vi "main.vi"() -> ()   [LabVIEW 2013]
uses:
  <vilib>/userdefined/High Color/IMAQdx.ctl
  <vilib>/Analysis/baseanly.llb/Mean (DBL).vi
  <vilib>/DAQmx/read.llb/DAQmx Read (Analog 1D Wfm NChan NSamp).vi
  <vilib>/measure/mascope.llb/Amplitude and Levels 1 chan.vi
  <vilib>/measure/mamon.llb/Trigger Detection for 1 Channel.vi
  <vilib>/Waveform/WDTOps.llb/WDT Append Waveforms DBL.vi
  <vilib>/DAQmx/miscellaneous.llb/DAQmx Fill In Error Info.vi
  <vilib>/measure/NI_MAPro.lvlib
  <vilib>/Analysis/NI_AALBase.lvlib
  <vilib>/vision/driver/NI_Vision_Acquisition_Software.lvlib
panel:
  in  "탭 컨트롤":T1(tab)
  out "웨이브폼 차트 2":dbl(graph)
  in  "reset":bool
  out "right":dbl(slide) scale=0.0..0.5
  out "left":dbl(slide)
  out "rear":dbl(slide) scale=0.0..0.5
  out "front":dbl(slide)
  out "trigger":bool
  in  "Force cal val":bool
  out "Triggered Force graph":waveform(dbl)(graph)={"t0"=timestamp(0 s since 1904-01-01), "dt"=0.00062, "Y"=array[3100 elements]}
  out "bonding force":dbl=1.1386680148675508 caption="Bonding force (kg)" format="%.3f"
  out "Bondtime":dbl=0.5053000000000001 caption="Bonding time" format="%.3f"
  out "vacum":dbl=1.2177873383633695 format="%#_3f"
  out "Heater temp":dbl=nan format="%0.2f"
  out "2":dbl(slide)
  out "슬라이드":dbl(slide)
  out "슬라이드 2":dbl(slide) scale=0.0..1.0
  out "슬라이드 3":dbl(slide) scale=0.0..1.0
  out "XY 그래프":cluster{dbl[], dbl[]}(graph)
  out "vaccum 차트 3":waveform(dbl)(graph)={"t0"=timestamp(3477442777.176875 s since 1904-01-01), "dt"=0.01, "Y"=[0.9261417940939543, 0.9261417940939543, 0.9261417940939543, 0.9261417940939543, 0.9261417940939543, 0.9261417940939543, 0.9261417940939543, 0.9261417940939543, 0.9261417940939543, 0.9261417940939543], "attributes"=variant("NI_ChannelName"=variant(string "전압"), "NI_UnitDescription"=variant(string "Volts"))}
  out "Force raw chart":waveform(dbl)[](graph)=[{"t0"=timestamp(3477442777.13187 s since 1904-01-01), "dt"=0.00062, "Y"=[-1.6112136636470233e-05, -8.569886798010926e-06, -1.9875060209823524e-07, 2.38297423695265e-06, -2.5658168581669667e-06, -1.772821098699811e-06, -4.127955201515539e-06, 6.359857628775875e-07, 4.928880013384412e-07, -3.030881455329775e-06, -1.6476111269731543e-06, -3.5257574105908386e-06, 3.9272455815972755e-06, 4.1657435117466915e-06, 1.9357923056845556e-06, -8.873963893666015e-06, -7.478785108954976e-06, 2.961286460921625e-07, 1.4110617831093333e-07, -1.8980310390713461e-06, 1.6734457588159683e-06, -1.091306434532689e-05, -1.0513727362142483e-06, -6.190924313818898e-06, -1.2540761368932031e-05, -2.1656959207560037e-05, -7.4907097304474685e-06, -3.2872630354662113e-06, -7.950263527933837e-08, -5.964355867846931e-06, -2.4107952296524134e-06, -3.7881010918357573e-06, 2.609546568115507e-06, 1.715182700246618e-06, -5.290612250873919e-06, -6.512889823589868e-06, -3.120361442334684e-07, 5.578846081749961e-06, 7.045614998740958e-06, -1.4627773018794912e-06, -7.937882831116044e-06, -2.595628704294203e-06, 1.2799261966089874e-06, 3.3190306855961753e-07, -3.4363220332503078e-06, -9.953137975658443e-06, 2.3591245238553327e-06, -1.0871470597100204e-06, 8.685197127258367e-07, -7.478785108954976e-06, -8.659321257106097e-06, -4.879210834785539e-06, -3.710590473067321e-06, -4.771888670569855e-06, -1.2516912366543758e-05, -5.576804340679935e-06, -6.274396873296863e-06, -8.546139112344271e-07, 2.2696881098723825e-06, -3.585380986597095e-06, -7.890184386099151e-06, 4.034519211733817e-07, 2.055040781583931e-06, 3.3071514956147953e-06, -2.7625750097582926e-06, -6.900440625190667e-06, 4.2909549706155075e-06, 9.830102788370948e-06, 3.032879356729265e-06, 4.088231671969834e-06, -9.488079817087242e-06, -5.111742111559042e-06, 2.567809552028929e-06, -4.688415860253707e-06, -1.833603522524735e-05, -9.50012139076079e-07, 3.3250388142463035e-06, -2.6135158111173114e-06, -6.769269618278701e-06, -2.0929577385222132e-05, -7.305878065355784e-06, -1.8562943957647073e-06, -3.090505090348801e-06, -3.5257574105908386e-06, -4.932871908254762e-06, -1.033522309183479e-07, -4.169691655199052e-06, 1.94771715199473e-06, -5.254838228130094e-06, -5.147516144541169e-06, 1.2978134427175586e-06, 9.126526251121246e-06, 1.5422725370008507e-06, -4.688415860253707e-06, -2.005353820147982e-06, 4.4518875659287035e-07, 1.7688444872052448e-06, -1.1229213806461855e-06, -6.51885214588969e-06, -1.4490413466475015e-05], "attributes"=variant("NI_ChannelName"=variant(string "변형률_0"), "NI_UnitDescription"=variant(string "Strain"))}, {"t0"=timestamp(3477442777.13187 s since 1904-01-01), "dt"=0.00062, "Y"=[-1.5926450874775857e-06, 1.7934307923881257e-06, -2.236473822173629e-06, -4.09045749208906e-06, -3.881810155491518e-06, 1.7218937409129746e-06, 3.9872386740088464e-06, 1.7192680555871353e-07, 2.2286147427125606e-06, -1.3005373326004466e-06, 3.456670124526979e-06, 8.523920832607e-06, 5.322604705970085e-06, 3.104945216654824e-06, 2.639953345335169e-06, 6.449322569493326e-06, 1.898110120282012e-07, -2.9306233811443237e-07, -7.929552945691535e-06, 2.53892933758521e-05, 6.6698972632327115e-06, 5.113953528386892e-06, 2.425341858268832e-06, -5.911320745626876e-07, -2.8385721664852527e-06, 1.0303694376600552e-06, -3.2286931975534613e-07, -4.793896442446842e-06, -2.7789585013682837e-06, -2.254357941858881e-06, 4.482039064584e-06, 3.188405341896096e-06, 2.890333530003795e-06, 1.5370897386411374e-06, 1.3224787249476363e-06, 5.0603003825103886e-06, 4.470116157849115e-06, 2.0378491288205883e-06, 3.087060905915481e-06, 4.237619533343155e-06, 6.22874797305966e-06, 2.4551490037417866e-06, 8.455656909807571e-07, -1.976799849226179e-07, -2.862417630541878e-06, 5.030493081733363e-06, 2.8068734545164028e-06, -7.640124402846258e-07, -2.105323591603382e-06, 2.3750223240719277e-07, 6.884510572159387e-06, -7.878580032793122e-07, -5.163499562134611e-06, -6.391533772034915e-06, -2.6835766223972933e-06, 4.684728522578421e-06, 2.885317683250044e-08, -1.2826531787987904e-06, -2.8206880676963555e-06, 3.7726266086577194e-06, 6.7414350226397595e-06, 3.3195569954219583e-06, 2.017338166964026e-07, 2.7114905281608864e-06, 3.40301715648635e-06, 9.60891530636603e-06, -7.029395011258529e-06, 2.153804825353152e-05, 1.1194680695472973e-05, -9.786224662971449e-07, 8.702765913475292e-06, -2.558387878634849e-06, -5.911320745626876e-07, -2.4272377325028147e-06, 2.8307191889483254e-06, 5.656446771208991e-06, 1.9901577367198323e-06, -2.2960875519699664e-06, -4.656785538247539e-06, -2.898185824494624e-06, 7.501831387741804e-07, -3.983153158427838e-06, -1.610529230191517e-06, -2.8028039682679484e-06, 4.458193251398366e-06, 9.171026170763248e-07, 3.748780829304955e-06, 1.9577241432685033e-07, 3.206289656260379e-06, 2.0974633753433343e-06, 7.442217298655735e-07, 6.548006047634227e-07, -1.8489844052503307e-06, 3.7964723891478954e-06, 8.0470009297029e-06, 2.5863004649327575e-06, 1.1674819390124968e-06, 3.150004752252312e-07, 3.188405341896096e-06, 5.7637531966593845e-06], "attributes"=variant("NI_ChannelName"=variant(string "변형률_1"), "NI_UnitDescription"=variant(string "Strain"))}, {"t0"=timestamp(3477442777.13187 s since 1904-01-01), "dt"=0.00062, "Y"=[-9.774144215970737e-06, -5.761376757146625e-06, 5.947220028941115e-07, -3.8056626676763385e-06, -7.275857412313684e-06, 3.1765375395588494e-06, -3.1557437920494864e-06, -3.000717146469372e-06, 7.974506851273759e-07, -1.8618660842482212e-06, -1.4862235419361472e-06, -6.721343374039278e-06, 8.62045556081355e-06, -3.294812422418737e-07, 2.115189123215763e-06, -2.3030966465335333e-06, -5.773301819593379e-06, -1.1940569250260916e-06, -5.171085810533189e-06, -2.538875015539028e-08, 3.6814298472928053e-07, -8.939395837287375e-06, 2.401395215885246e-06, -4.646382161832467e-06, -7.311632490439199e-06, -2.205074690463858e-05, -3.5313850800753163e-06, -4.425767963291082e-06, -3.6148608835335274e-06, -1.677026138378287e-06, -2.5952626153941553e-06, 3.26404755740087e-07, -2.601225184409818e-06, 1.4056372250135049e-06, -1.1753684800069817e-05, -4.914696596438629e-06, 5.808765257422834e-08, 6.318857576908811e-06, 3.9934195965366175e-06, 5.03688401927312e-06, -6.059503232998047e-06, -5.4811377077647035e-06, 1.3937119916306282e-06, -7.055244373975443e-06, 7.318619848217363e-07, -1.718764196644247e-06, 4.814324809771893e-07, -1.0119968136008337e-05, 1.984011385493666e-06, -1.0131893094502119e-05, -1.0251142663796572e-05, -3.865288210289022e-06, -6.06546576070178e-06, -6.995619211769368e-06, 2.1867406310243084e-06, -1.0119968136008337e-05, -8.080796051007461e-06, -1.7962777241804084e-06, -1.2536827790775241e-06, 1.4771886312832808e-06, 2.2284790153078483e-06, -6.190678826058288e-06, -1.7068390374955085e-06, 1.4593007787556523e-06, 5.024958699283277e-06, 2.1927032571370627e-06, 5.589463616211063e-07, -4.831221009990731e-06, -8.959275481128778e-07, 3.421005752440379e-06, 3.987456948949547e-06, -4.205153667407975e-06, -9.674786147839707e-07, -5.212823577128643e-06, -1.6183772832057885e-05, 9.294241431321112e-06, -3.257107342016943e-06, -4.473468338791205e-06, -1.0316729914785664e-05, -1.128265025116678e-05, -1.0650628513704086e-05, -4.65234470638786e-06, -2.362722368329657e-06, -7.230124280525015e-07, 7.139741589589915e-07, -2.326946936105031e-06, -1.5277486145651072e-05, 1.411599841811428e-06, -3.3703959911923048e-06, -5.7852268817560655e-06, 2.17481537901177e-06, 2.5325730631100896e-06, -1.981117625965015e-06, -2.3209843638189005e-06, -2.6191128910294843e-06, 9.047776678219688e-07, -6.514613263977364e-07, -9.495908490762017e-07, 5.470211484321648e-07, -1.2970025127066287e-05], "attributes"=variant("NI_ChannelName"=variant(string "변형률_2"), "NI_UnitDescription"=variant(string "Strain"))}, {"t0"=timestamp(3477442777.13187 s since 1904-01-01), "dt"=0.00062, "Y"=[-7.598292136517871e-06, -3.990960943167142e-06, -3.961148180242939e-06, 8.446924425047726e-07, -3.865747326939833e-06, -6.459578537381319e-07, -5.028556181360945e-07, -4.313044849763774e-07, -2.0352399287900154e-06, -2.1843042998043006e-06, 2.317459299605134e-06, 2.520188680335006e-06, 1.8642998046072807e-06, 3.1998303138911986e-07, -2.3810692014959805e-06, 1.1129194138591358e-07, -3.919410309162601e-06, -4.181762583788524e-06, -2.9177003579997263e-06, -2.887887531081505e-06, 8.147893563887326e-08, -5.910899132064934e-06, 5.841384650575335e-06, -7.771348670609545e-07, -9.965402760758176e-06, -5.064219224553743e-06, -1.0078689889986319e-05, -8.14684269941332e-06, -4.8913055460130025e-06, -2.0292773530250545e-06, -2.5003206193811262e-06, -4.098286874975869e-06, -3.305266946174274e-06, -4.038661360148547e-06, -2.4228072009909966e-06, -2.1366037059148034e-06, -4.217537883299131e-06, -1.2183663865814867e-06, -2.5062831895288145e-06, 1.1725454274867201e-07, 3.9571845882479464e-06, -1.8087543828407676e-07, -4.0803992212742764e-06, -1.2064412154978175e-06, -5.839348772806825e-06, -1.8563626249113895e-06, -5.213282692541838e-06, -3.1800531582297593e-06, -1.8742503581789873e-06, -3.8360372384809986e-07, -4.181762583788524e-06, -6.0420747641119605e-06, -4.050586463682811e-06, -3.531844197032469e-06, -2.3452937705841765e-06, -7.1034036122986465e-06, -1.32569291353597e-06, -1.6953729967054738e-06, -1.7549987909737935e-06, -2.8699998340773e-06, -4.825717583337447e-06, -2.46454519700197e-06, 1.1964865605783791e-06, 3.378708431566748e-07, 2.889871880335409e-06, 2.0908795007679327e-06, -1.0514139655274806e-06, 5.501512595474361e-06, -3.376817668063878e-06, -4.819755040849376e-06, -1.5701588055974375e-06, -5.064219224553743e-06, -8.904240781442745e-07, 4.028736359651292e-06, -4.1996502338637966e-06, -6.918565604118794e-06, -3.996923495538705e-06, -3.3648925484600175e-06, -1.3024146240405366e-05, -8.289942747279497e-06, -7.061666003521132e-06, -5.165582387620764e-06, -6.823165315097408e-06, -1.0633391403086943e-06, -1.9517638616103747e-06, -5.255020455614867e-06, -2.4705077675762867e-06, -1.7491284040547266e-07, -3.1919782822420984e-06, -2.858074702385669e-06, -1.9815767443457687e-06, 2.317459299605134e-06, 3.927371353185168e-06, 3.665014961285459e-06, 2.186281508816372e-06, -1.0096758515535991e-06, -1.5522710614508004e-06, -6.507151727700881e-06, -2.16045400342839e-06, -2.893850096607393e-06], "attributes"=variant("NI_ChannelName"=variant(string "변형률_3"), "NI_UnitDescription"=variant(string "Strain"))}]
  in  "display":bool=TRUE
  out "vacum 2":dbl=0.9261417940939543 format="%#_3f"
  out "x-y 2":u32=56
  out "x-y":u32=99
  out "Filtered force 차트":waveform(dbl)[](graph)
  out "Force raw graph":waveform(dbl)[](graph)=[{"t0"=timestamp(3477442777.13187 s since 1904-01-01), "dt"=0.00062, "Y"=[-1.6112136636470233e-05, -8.569886798010926e-06, -1.9875060209823524e-07, 2.38297423695265e-06, -2.5658168581669667e-06, -1.772821098699811e-06, -4.127955201515539e-06, 6.359857628775875e-07, 4.928880013384412e-07, -3.030881455329775e-06, -1.6476111269731543e-06, -3.5257574105908386e-06, 3.9272455815972755e-06, 4.1657435117466915e-06, 1.9357923056845556e-06, -8.873963893666015e-06, -7.478785108954976e-06, 2.961286460921625e-07, 1.4110617831093333e-07, -1.8980310390713461e-06, 1.6734457588159683e-06, -1.091306434532689e-05, -1.0513727362142483e-06, -6.190924313818898e-06, -1.2540761368932031e-05, -2.1656959207560037e-05, -7.4907097304474685e-06, -3.2872630354662113e-06, -7.950263527933837e-08, -5.964355867846931e-06, -2.4107952296524134e-06, -3.7881010918357573e-06, 2.609546568115507e-06, 1.715182700246618e-06, -5.290612250873919e-06, -6.512889823589868e-06, -3.120361442334684e-07, 5.578846081749961e-06, 7.045614998740958e-06, -1.4627773018794912e-06, -7.937882831116044e-06, -2.595628704294203e-06, 1.2799261966089874e-06, 3.3190306855961753e-07, -3.4363220332503078e-06, -9.953137975658443e-06, 2.3591245238553327e-06, -1.0871470597100204e-06, 8.685197127258367e-07, -7.478785108954976e-06, -8.659321257106097e-06, -4.879210834785539e-06, -3.710590473067321e-06, -4.771888670569855e-06, -1.2516912366543758e-05, -5.576804340679935e-06, -6.274396873296863e-06, -8.546139112344271e-07, 2.2696881098723825e-06, -3.585380986597095e-06, -7.890184386099151e-06, 4.034519211733817e-07, 2.055040781583931e-06, 3.3071514956147953e-06, -2.7625750097582926e-06, -6.900440625190667e-06, 4.2909549706155075e-06, 9.830102788370948e-06, 3.032879356729265e-06, 4.088231671969834e-06, -9.488079817087242e-06, -5.111742111559042e-06, 2.567809552028929e-06, -4.688415860253707e-06, -1.833603522524735e-05, -9.50012139076079e-07, 3.3250388142463035e-06, -2.6135158111173114e-06, -6.769269618278701e-06, -2.0929577385222132e-05, -7.305878065355784e-06, -1.8562943957647073e-06, -3.090505090348801e-06, -3.5257574105908386e-06, -4.932871908254762e-06, -1.033522309183479e-07, -4.169691655199052e-06, 1.94771715199473e-06, -5.254838228130094e-06, -5.147516144541169e-06, 1.2978134427175586e-06, 9.126526251121246e-06, 1.5422725370008507e-06, -4.688415860253707e-06, -2.005353820147982e-06, 4.4518875659287035e-07, 1.7688444872052448e-06, -1.1229213806461855e-06, -6.51885214588969e-06, -1.4490413466475015e-05], "attributes"=variant("NI_ChannelName"=variant(string "변형률_0"), "NI_UnitDescription"=variant(string "Strain"))}, {"t0"=timestamp(3477442777.13187 s since 1904-01-01), "dt"=0.00062, "Y"=[-1.5926450874775857e-06, 1.7934307923881257e-06, -2.236473822173629e-06, -4.09045749208906e-06, -3.881810155491518e-06, 1.7218937409129746e-06, 3.9872386740088464e-06, 1.7192680555871353e-07, 2.2286147427125606e-06, -1.3005373326004466e-06, 3.456670124526979e-06, 8.523920832607e-06, 5.322604705970085e-06, 3.104945216654824e-06, 2.639953345335169e-06, 6.449322569493326e-06, 1.898110120282012e-07, -2.9306233811443237e-07, -7.929552945691535e-06, 2.53892933758521e-05, 6.6698972632327115e-06, 5.113953528386892e-06, 2.425341858268832e-06, -5.911320745626876e-07, -2.8385721664852527e-06, 1.0303694376600552e-06, -3.2286931975534613e-07, -4.793896442446842e-06, -2.7789585013682837e-06, -2.254357941858881e-06, 4.482039064584e-06, 3.188405341896096e-06, 2.890333530003795e-06, 1.5370897386411374e-06, 1.3224787249476363e-06, 5.0603003825103886e-06, 4.470116157849115e-06, 2.0378491288205883e-06, 3.087060905915481e-06, 4.237619533343155e-06, 6.22874797305966e-06, 2.4551490037417866e-06, 8.455656909807571e-07, -1.976799849226179e-07, -2.862417630541878e-06, 5.030493081733363e-06, 2.8068734545164028e-06, -7.640124402846258e-07, -2.105323591603382e-06, 2.3750223240719277e-07, 6.884510572159387e-06, -7.878580032793122e-07, -5.163499562134611e-06, -6.391533772034915e-06, -2.6835766223972933e-06, 4.684728522578421e-06, 2.885317683250044e-08, -1.2826531787987904e-06, -2.8206880676963555e-06, 3.7726266086577194e-06, 6.7414350226397595e-06, 3.3195569954219583e-06, 2.017338166964026e-07, 2.7114905281608864e-06, 3.40301715648635e-06, 9.60891530636603e-06, -7.029395011258529e-06, 2.153804825353152e-05, 1.1194680695472973e-05, -9.786224662971449e-07, 8.702765913475292e-06, -2.558387878634849e-06, -5.911320745626876e-07, -2.4272377325028147e-06, 2.8307191889483254e-06, 5.656446771208991e-06, 1.9901577367198323e-06, -2.2960875519699664e-06, -4.656785538247539e-06, -2.898185824494624e-06, 7.501831387741804e-07, -3.983153158427838e-06, -1.610529230191517e-06, -2.8028039682679484e-06, 4.458193251398366e-06, 9.171026170763248e-07, 3.748780829304955e-06, 1.9577241432685033e-07, 3.206289656260379e-06, 2.0974633753433343e-06, 7.442217298655735e-07, 6.548006047634227e-07, -1.8489844052503307e-06, 3.7964723891478954e-06, 8.0470009297029e-06, 2.5863004649327575e-06, 1.1674819390124968e-06, 3.150004752252312e-07, 3.188405341896096e-06, 5.7637531966593845e-06], "attributes"=variant("NI_ChannelName"=variant(string "변형률_1"), "NI_UnitDescription"=variant(string "Strain"))}, {"t0"=timestamp(3477442777.13187 s since 1904-01-01), "dt"=0.00062, "Y"=[-9.774144215970737e-06, -5.761376757146625e-06, 5.947220028941115e-07, -3.8056626676763385e-06, -7.275857412313684e-06, 3.1765375395588494e-06, -3.1557437920494864e-06, -3.000717146469372e-06, 7.974506851273759e-07, -1.8618660842482212e-06, -1.4862235419361472e-06, -6.721343374039278e-06, 8.62045556081355e-06, -3.294812422418737e-07, 2.115189123215763e-06, -2.3030966465335333e-06, -5.773301819593379e-06, -1.1940569250260916e-06, -5.171085810533189e-06, -2.538875015539028e-08, 3.6814298472928053e-07, -8.939395837287375e-06, 2.401395215885246e-06, -4.646382161832467e-06, -7.311632490439199e-06, -2.205074690463858e-05, -3.5313850800753163e-06, -4.425767963291082e-06, -3.6148608835335274e-06, -1.677026138378287e-06, -2.5952626153941553e-06, 3.26404755740087e-07, -2.601225184409818e-06, 1.4056372250135049e-06, -1.1753684800069817e-05, -4.914696596438629e-06, 5.808765257422834e-08, 6.318857576908811e-06, 3.9934195965366175e-06, 5.03688401927312e-06, -6.059503232998047e-06, -5.4811377077647035e-06, 1.3937119916306282e-06, -7.055244373975443e-06, 7.318619848217363e-07, -1.718764196644247e-06, 4.814324809771893e-07, -1.0119968136008337e-05, 1.984011385493666e-06, -1.0131893094502119e-05, -1.0251142663796572e-05, -3.865288210289022e-06, -6.06546576070178e-06, -6.995619211769368e-06, 2.1867406310243084e-06, -1.0119968136008337e-05, -8.080796051007461e-06, -1.7962777241804084e-06, -1.2536827790775241e-06, 1.4771886312832808e-06, 2.2284790153078483e-06, -6.190678826058288e-06, -1.7068390374955085e-06, 1.4593007787556523e-06, 5.024958699283277e-06, 2.1927032571370627e-06, 5.589463616211063e-07, -4.831221009990731e-06, -8.959275481128778e-07, 3.421005752440379e-06, 3.987456948949547e-06, -4.205153667407975e-06, -9.674786147839707e-07, -5.212823577128643e-06, -1.6183772832057885e-05, 9.294241431321112e-06, -3.257107342016943e-06, -4.473468338791205e-06, -1.0316729914785664e-05, -1.128265025116678e-05, -1.0650628513704086e-05, -4.65234470638786e-06, -2.362722368329657e-06, -7.230124280525015e-07, 7.139741589589915e-07, -2.326946936105031e-06, -1.5277486145651072e-05, 1.411599841811428e-06, -3.3703959911923048e-06, -5.7852268817560655e-06, 2.17481537901177e-06, 2.5325730631100896e-06, -1.981117625965015e-06, -2.3209843638189005e-06, -2.6191128910294843e-06, 9.047776678219688e-07, -6.514613263977364e-07, -9.495908490762017e-07, 5.470211484321648e-07, -1.2970025127066287e-05], "attributes"=variant("NI_ChannelName"=variant(string "변형률_2"), "NI_UnitDescription"=variant(string "Strain"))}, {"t0"=timestamp(3477442777.13187 s since 1904-01-01), "dt"=0.00062, "Y"=[-7.598292136517871e-06, -3.990960943167142e-06, -3.961148180242939e-06, 8.446924425047726e-07, -3.865747326939833e-06, -6.459578537381319e-07, -5.028556181360945e-07, -4.313044849763774e-07, -2.0352399287900154e-06, -2.1843042998043006e-06, 2.317459299605134e-06, 2.520188680335006e-06, 1.8642998046072807e-06, 3.1998303138911986e-07, -2.3810692014959805e-06, 1.1129194138591358e-07, -3.919410309162601e-06, -4.181762583788524e-06, -2.9177003579997263e-06, -2.887887531081505e-06, 8.147893563887326e-08, -5.910899132064934e-06, 5.841384650575335e-06, -7.771348670609545e-07, -9.965402760758176e-06, -5.064219224553743e-06, -1.0078689889986319e-05, -8.14684269941332e-06, -4.8913055460130025e-06, -2.0292773530250545e-06, -2.5003206193811262e-06, -4.098286874975869e-06, -3.305266946174274e-06, -4.038661360148547e-06, -2.4228072009909966e-06, -2.1366037059148034e-06, -4.217537883299131e-06, -1.2183663865814867e-06, -2.5062831895288145e-06, 1.1725454274867201e-07, 3.9571845882479464e-06, -1.8087543828407676e-07, -4.0803992212742764e-06, -1.2064412154978175e-06, -5.839348772806825e-06, -1.8563626249113895e-06, -5.213282692541838e-06, -3.1800531582297593e-06, -1.8742503581789873e-06, -3.8360372384809986e-07, -4.181762583788524e-06, -6.0420747641119605e-06, -4.050586463682811e-06, -3.531844197032469e-06, -2.3452937705841765e-06, -7.1034036122986465e-06, -1.32569291353597e-06, -1.6953729967054738e-06, -1.7549987909737935e-06, -2.8699998340773e-06, -4.825717583337447e-06, -2.46454519700197e-06, 1.1964865605783791e-06, 3.378708431566748e-07, 2.889871880335409e-06, 2.0908795007679327e-06, -1.0514139655274806e-06, 5.501512595474361e-06, -3.376817668063878e-06, -4.819755040849376e-06, -1.5701588055974375e-06, -5.064219224553743e-06, -8.904240781442745e-07, 4.028736359651292e-06, -4.1996502338637966e-06, -6.918565604118794e-06, -3.996923495538705e-06, -3.3648925484600175e-06, -1.3024146240405366e-05, -8.289942747279497e-06, -7.061666003521132e-06, -5.165582387620764e-06, -6.823165315097408e-06, -1.0633391403086943e-06, -1.9517638616103747e-06, -5.255020455614867e-06, -2.4705077675762867e-06, -1.7491284040547266e-07, -3.1919782822420984e-06, -2.858074702385669e-06, -1.9815767443457687e-06, 2.317459299605134e-06, 3.927371353185168e-06, 3.665014961285459e-06, 2.186281508816372e-06, -1.0096758515535991e-06, -1.5522710614508004e-06, -6.507151727700881e-06, -2.16045400342839e-06, -2.893850096607393e-06], "attributes"=variant("NI_ChannelName"=variant(string "변형률_3"), "NI_UnitDescription"=variant(string "Strain"))}]
  out "Filtered force 그래프":waveform(dbl)[](graph)
  out "Strain front":dbl(graph)=0.21080623907694704
  out "Strain left":dbl(graph)=0.40238302318753916
  out "Strain rear":dbl(graph)=0.4140902820131476
  out "Strain right":dbl(graph)=0.09497703213784708
  out "강도 그래프 2":dbl[][](graph)=[[nan, nan, nan, nan], [nan, nan, nan, nan]]
  out "Image":T2(plugin-control)
  out "error out":errorcluster={"status"=FALSE, "code"=-1074360308, "source"=""}
  out "Heater temp 2":dbl=nan caption="Heater temp" format="%0.2f"
  out "data":dynamicdata(graph)=[{"t0"=timestamp(3477442777.176875 s since 1904-01-01), "dt"=0.01, "Y"=[0.9261417940939543, 0.9261417940939543, 0.9261417940939543, 0.9261417940939543, 0.9261417940939543, 0.9261417940939543, 0.9261417940939543, 0.9261417940939543, 0.9261417940939543, 0.9261417940939543], "attributes"=variant("NI_ChannelName"=variant(string "전압"), "NI_UnitDescription"=variant(string "Volts"))}] caption="데이터"
  in  "bonding time trigger edge level":dbl=0.5 format="%#_13g"
  out "front mean":dbl=0.24100886710135544 format="%0.2f"
  out "left mean":dbl=0.5329196805184643 format="%0.2f"
  out "rear mean 3":dbl=0.3563222576715275 caption="rear mean" format="%0.2f"
  out "right mean 4":dbl=0.1826222935697912 caption="right mean" format="%0.2f"
  in  "Force trigger minimum level":dbl=0.5 format="%#_13g"
  in  "state settings":T3={"method"=enum."histogram", "histogram size"=512, "histogram method"=enum."mode", "reserved"=1.0} caption="상태 셋팅" {"reserved" format="%0.2f"}
  out "level1 4":dbl=0.09497703213784708 caption="right F" format="%.2g"
  out "level1 3":dbl=0.4140902820131476 caption="rear F" format="%.2g"
  out "level1 2":dbl=0.40238302318753916 caption="left F" format="%.2g"
  out "level1":dbl=0.21080623907694704 caption="front F" format="%.2g"
  in  "Lower Cut-Off":dbl=20.0 caption="하위 컷오프"
  out "웨이브폼 차트":waveform(dbl)[](graph)
  out "force offset":dbl
  out "trigger location 2":dbl=1.84016 caption="트리거 falling" format="%#.3f"
  out "trigger location":dbl=1.33486 caption="트리거 rising" format="%#.3f"
  out "strain high level mean":T4={"mean"=0.24100886710135544, "mean"=0.5329196805184643, "mean"=0.3563222576715275, "mean"=0.1826222935697912}
  in  "정지":bool=TRUE
  # "Die Attach Machine Monitoring"
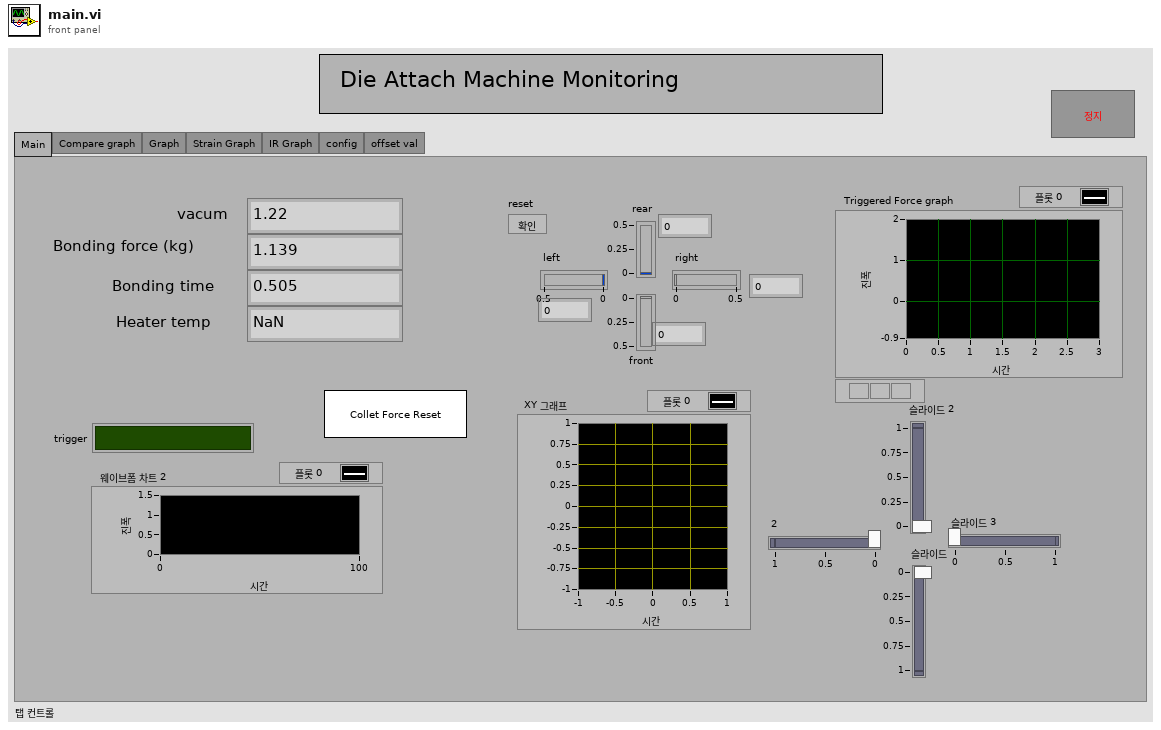
[diagram p1: front panel]
types:
  T1 = enum32{"Main", "Compare graph", "Graph", "Strain Graph", "IR Graph", "config", "offset val"}
  T2 = typedef "IMAQ Image.ctl" = refnum<image>
  T3 = cluster{"method":enum32{"histogram", "peak", "auto select"}, "histogram size":i32, "histogram method":enum16{"mode"}, "reserved":dbl}
  T4 = cluster{"mean":dbl, "mean":dbl, "mean":dbl, "mean":dbl}
  T5 = typedef "IMAQdx.ctl" = refnum<k21>
  T6 = cluster{"Global Rectangle":i32[], "Contours":cluster{"Contour Type":u32, "ROI Type":u32, "Points":i32[]}[]}
  T7 = cluster{"high state level":dbl, "high state level":dbl, "high state level":dbl, "high state level":dbl}
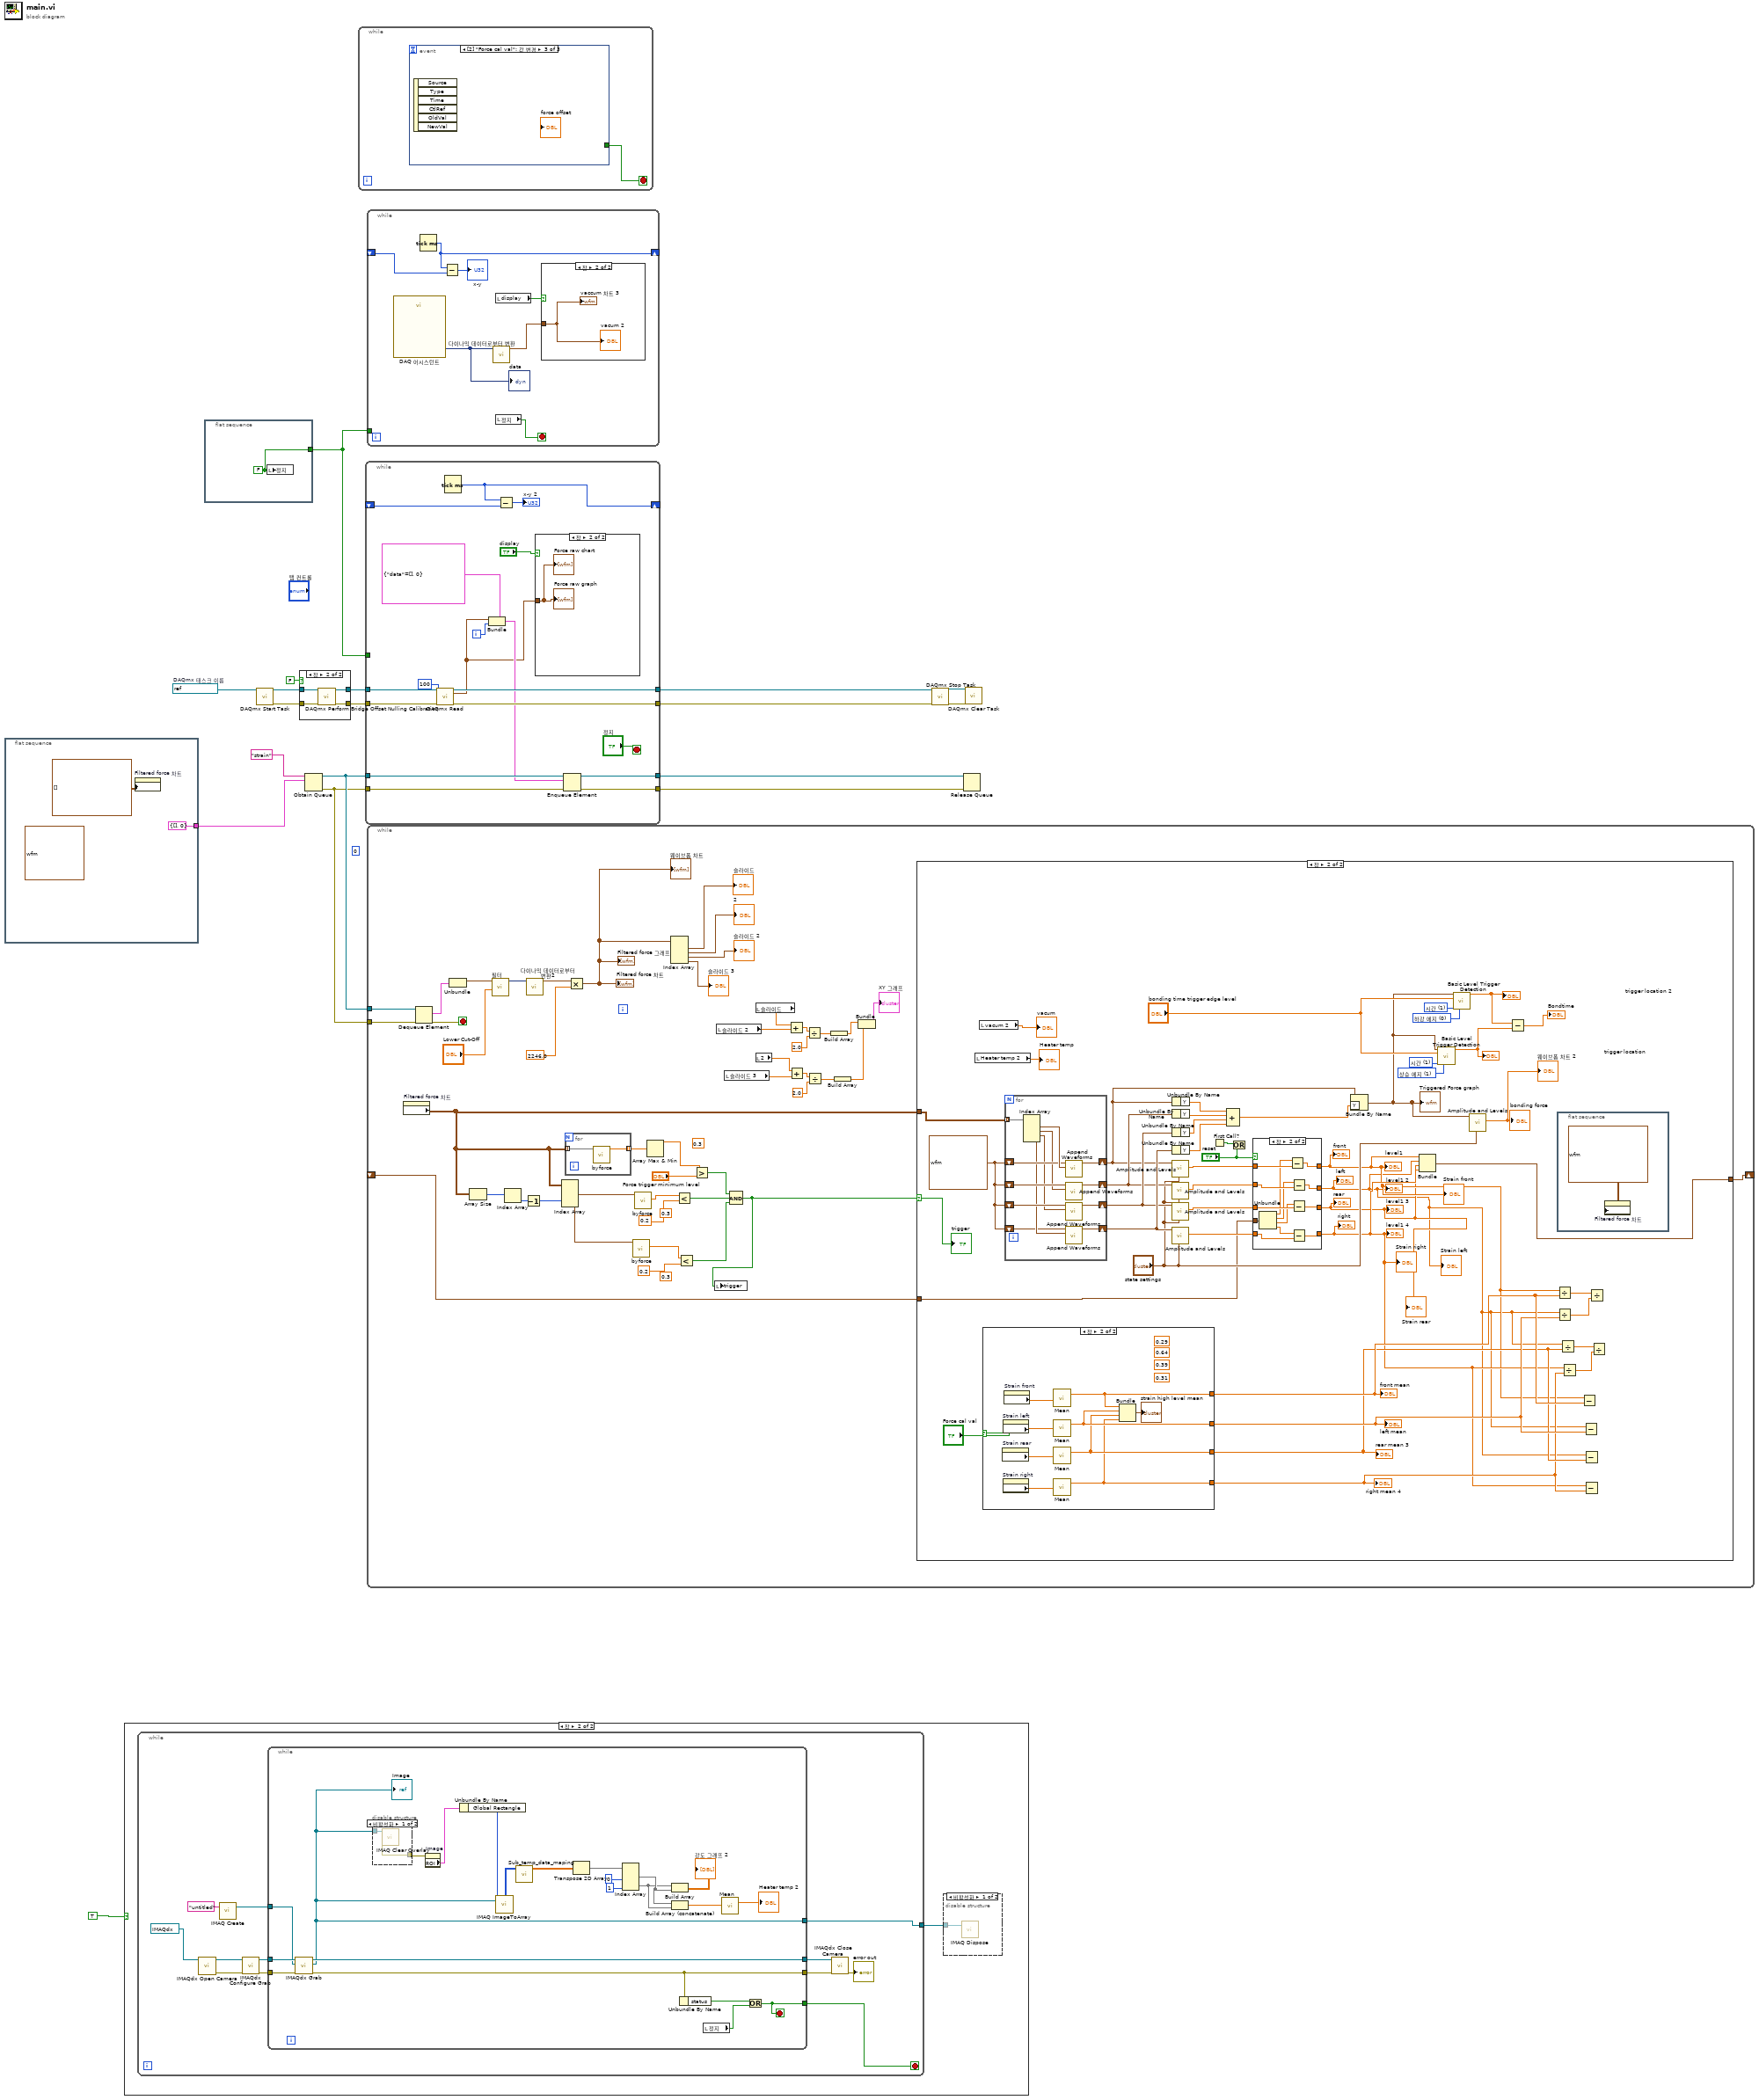
[diagram p0: block diagram]
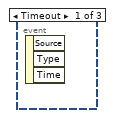
[diagram p6: hidden frame]
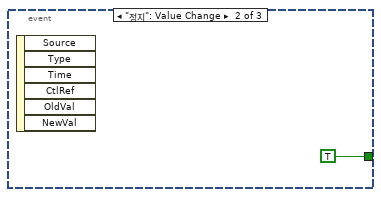
[diagram p7: hidden frame]
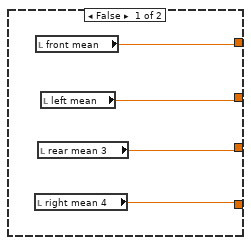
[diagram p10: hidden frame]
diagram:
  (unwired) 0 ("y")
  w16 = refnum<k21> "9237_task"  # DAQmx 태스크 이름
  n1 = flat-sequence {
    tunnel: [cluster{"data":waveform(dbl)[], i32} {"data"=[], 0}] -> w7
    frame #0 {
      (unwired) waveform(dbl) {"t0"=timestamp(0 s since 1904-01-01), "dt"=1.0, "Y"=[]} ("Waveform")
      n2 = property on="Filtered force 차트" class="WFChart (엄격한)"("History Data"=waveform(dbl)[][] [] ("히스토리 데이터")) -> ()  [unwired: 2 in, 2 out]
    }
  }
  n3 = case shown="참" TRUE {
    frame False {
    }
    frame True {
      n4 = while {
        tunnel: [w24] -> w21
        stop <- w23 stop-if-true
        n5 = call <vilib>:"IMAQdx Open Camera.vi"("Session In"=T5 "ssw") -> ("error out"=w30:errorcluster, "Session Out"=w33:T5)  [unwired: 9 in]
        n6 = call "IMAQ Create"("Image Name"="untitled") -> ("New Image"=w26:T2)  [unwired: 4 in, 1 out]
        n7 = call <vilib>:"IMAQdx Configure Grab.vi"("error in"=w30, "Session In"=w33) -> ("error out"=w29:errorcluster, "Session Out"=w32:T5)  [unwired: 8 in]
        n8 = while {
          tunnel: w32 -> [w55]
          tunnel: [w54] -> w31
          tunnel: w29 -> [w53]
          tunnel: [w51] -> w28
          tunnel: w26 -> [w52]
          tunnel: [w40] -> w24
          tunnel: [w35] -> w23
          stop <- w35 stop-if-true
          n9 = call <vilib>:"IMAQdx Grab.vi"("error in"=w53, "Image In"=w52, "Session In"=w55) -> ("error out"=w51:errorcluster, "Image Out"=w40:T2, "Session Out"=w54:T5)  [unwired: 5 in, 1 out]
          "Image" <- w40
          n10 = disable-structure shown="비활성화" {
            disable-tunnel: w40 -> [w57 _]
            disable-tunnel: [w56 _] -> w49
            frame Disabled {
              n11 = call "IMAQ Clear Overlay"("Image"=w57) -> ("error out"=w56:errorcluster)  [unwired: 9 in, 1 out]
            }
            frame Enabled {
            }
          }
          n12 = property on="Image" class="ImageControl"(error in=w49) -> ("ROI"=w48:T6)  [unwired: 1 in, 2 out]
          n13 = Unbundle By Name(w48) -> ("Global Rectangle"=w47:i32[])
          n14 = call "IMAQ ImageToArray"("Optional Rectangle"=w47, "Image"=w40) -> ("Image Pixels (U8)"=w46:u8[][])  [unwired: 2 in, 4 out]
          n15 = call "Sub_temp_data_maping.vi"("temp_data"=w46) -> ("mapping_temp"=w36:dbl[][])  [unwired: 10 in]
          n16 = Transpose 2D Array(2D array=w36) -> (transposed array=w42:dbl[][])
          n17 = Index Array(array=w42, index (col) #1=0 ("비활성화된 인덱스 (열)"), index (col) #2=1 ("비활성화된 인덱스 (열)")) -> (element #1=w39:dbl[], element #2=w38:dbl[])  [unwired: 2 in]
          n18 = Build Array(w38, w39) -> (→"강도 그래프 2":dbl[][])
          n19 = Build Array (concatenate)(w39, w38) -> (w37:dbl[])
          n20 = Unbundle By Name(w51) -> ("status"=w50:bool)
          n21 = local read "정지"() -> (w41:bool)
          n22 = call-poly <vilib>:"Mean.vi"("X"=w37) -> ("mean"=→"Heater temp 2":dbl)  [unwired: 1 out]
          n23 = Or(x=w50, y=w41) -> (x .or. y?=w35:bool)
        }
        n24 = call <vilib>:"IMAQdx Close Camera.vi"("error in"=w28, "Session In"=w31) -> ("error out"=→"error out":errorcluster)  [unwired: 9 in]
      }
      n25 = disable-structure shown="비활성화" {
        disable-tunnel: w21 -> [w58 _]
        frame Disabled {
          n26 = call "IMAQ Dispose"("Image"=w58) -> ()  [unwired: 5 in, 1 out]
        }
        frame Enabled {
        }
      }
    }
  }
  n27 = flat-sequence {
    tunnel: [w59] -> w13
    frame #0 {
      w59 = FALSE ("정지")
      n28 = local write "정지"(w59) -> ()
    }
  }
  n29 = call <vilib>:"DAQmx Start Task.vi"("task/channels in"=w16) -> ("task out"=w6:refnum<k21>, "error out"=w5:errorcluster)  [unwired: 13 in]
  n30 = case shown="참" FALSE {
    tunnel: w6 -> [w61 w65]
    tunnel: w5 -> [w60 w64]
    tunnel: [w60 w63] -> w4
    tunnel: [w61 w62] -> w3
    frame False {
    }
    frame True {
      n31 = call <vilib>:"DAQmx Perform Bridge Offset Nulling Calibration.vi"("task/channels in"=w65, "error in"=w64) -> ("task out"=w62:refnum<k21>, "error out"=w63:errorcluster)  [unwired: 12 in]
    }
  }
  n32 = Obtain Queue(name (unnamed)="strain" ("이름(이름없음)"), element data type=w7) -> (queue out=w11:refnum<queue>, error out=w9:errorcluster)  [unwired: 3 in, 1 out]
  n33 = while {
    stop <- w66 stop-if-true
    n34 = event shown="[2] \"Force cal val\": 값 변경" {
      selector: _ -> [_ _ _]
      dyn-events: _ -> [_ _ _]
      timeout: _ -> [_ _ _]
      tunnel: [_ TRUE _] -> w66
      event Timeout {
        n35 = event-data() -> ()  [unwired: 1 in, 3 out]
      }
      event "정지": Value Change {
        n36 = event-data() -> ()  [unwired: 1 in, 6 out]
      }
      event "Force cal val": Value Change {
        n37 = event-data() -> ()  [unwired: 1 in, 6 out]
      }
    }
  }
  n38 = while {
    tunnel: w4 -> [w85]
    tunnel: w3 -> [w84]
    tunnel: [w83] -> w18
    tunnel: [w82] -> w17
    tunnel: w13 -> [_]
    tunnel: w11 -> [w79]
    tunnel: [w78] -> w10
    tunnel: w9 -> [w77]
    tunnel: [w76] -> w8
    shift-right: [w71] -> _
    shift-left: _ -> [w72]
    i -> [w74]
    stop <- "정지" stop-if-true
    n39 = call-poly <vilib>:"DAQmx Read.vi"("task/channels in"=w84, "number of samples per channel"=100, "error in"=w85) -> ("task out"=w82:refnum<k21>, "data"=w69:waveform(dbl)[], "error out"=w83:errorcluster)  [unwired: 10 in]
    n40 = Tick Count (ms)() -> (millisecond timer value=w71:u32)
    n41 = Bundle(cluster=cluster{"data":waveform(dbl)[], i32} {"data"=[], 0}, "data"=w69, w74) -> (w73:cluster{"data":waveform(dbl)[], i32})
    n42 = Subtract(x=w71, y=w72) -> (x-y=→"x-y 2":u32)
    n43 = case shown="참" "display" {
      tunnel: w69 -> [_ w86]
      frame False {
      }
      frame True {
        "Force raw graph" <- w86
        "Force raw chart" <- w86
      }
    }
    n44 = Enqueue Element(queue=w79, element=w73, error in (no error)=w77) -> (queue out=w78:refnum<queue>, error out=w76:errorcluster)  [unwired: 1 in, 1 out]
  }
  n45 = while {
    tunnel: w13 -> [_]
    shift-right: [w92] -> _
    shift-left: _ -> [w91]
    stop <- w93 stop-if-true
    n46 = call "DAQ 어시스턴트"() -> ("data"=w89:dynamicdata)  [unwired: 16 in, 3 out]
    "data" <- w89
    n47 = Tick Count (ms)() -> (millisecond timer value=w92:u32)
    n48 = Subtract(x=w92, y=w91) -> (x-y=→"x-y":u32)
    n49 = call "다이나믹 데이터로부터 변환"("Dynamic Data Type"=w89) -> ("Waveform"=w88:waveform(dbl))  [unwired: 3 in]
    n50 = local read "정지"() -> (w93:bool)
    n51 = local read "display"() -> (w87:bool)
    n52 = case shown="참" w87 {
      tunnel: w88 -> [_ w94]
      frame False {
      }
      frame True {
        "vaccum 차트 3" <- w94
        "vacum 2" <- w94
      }
    }
  }
  n53 = while {
    tunnel: w11 -> [w140]
    tunnel: w9 -> [w139]
    shift-right: [w114] -> _
    shift-left: _ -> [w113]
    stop <- w138 stop-if-true
    (unwired) 0.3 ("y")
    (unwired) 0.3 ("y")
    (unwired) 0.3 ("y")
    n54 = property on="Filtered force 차트" class="WFChart (엄격한)"() -> ("History Data"=w123:waveform(dbl)[][])  [unwired: 2 in, 2 out]
    n55 = Dequeue Element(queue=w140, error in (no error)=w139) -> (element=w136:cluster{"data":waveform(dbl)[], i32}, error out=w138:errorcluster)  [unwired: 1 in, 2 out]
    n56 = Unbundle(w136) -> ("data"=w122:waveform(dbl)[])  [unwired: 1 out]
    n57 = Array Size(array=w123) -> (size(s)=w135:i32[])
    n58 = call "필터"("Lower Cut-Off"="Lower Cut-Off", "Signal"=w122) -> ("Filtered Signal"=w121:dynamicdata)  [unwired: 8 in, 1 out]
    n59 = Index Array(array=w135) -> (element=w134:i32)  [unwired: 1 in]
    n60 = Decrement(x=w134) -> (x-1=w133:i32)
    n61 = call "다이나믹 데이터로부터 변환2"("Dynamic Data Type"=w121) -> ("Array of Waveform"=w120:waveform(dbl)[])  [unwired: 3 in]
    n62 = Index Array(array=w123, index (row) #2=w133) -> (element #1=w132:waveform(dbl)[], element #2=w131:waveform(dbl)[])  [unwired: 3 in]
    n63 = for {
      tunnel: w123 -> [w233] mode=indexing
      tunnel: [w232] -> w128 mode=indexing
      n64 = call "byforce.vi"("History Data"=w233) -> ("mean"=w232:dbl)  [unwired: 8 in, 2 out]
    }
    n65 = Multiply(x=w120, y=2246.0) -> (x*y=w95:waveform(dbl)[])
    "Filtered force 그래프" <- w95
    "Filtered force 차트" <- w95
    "웨이브폼 차트" <- w95
    n66 = call "byforce.vi"("History Data"=w131) -> ("max"=w118:dbl)  [unwired: 8 in, 2 out]
    n67 = call "byforce.vi"("History Data"=w132) -> ("max"=w119:dbl)  [unwired: 8 in, 2 out]
    n68 = Array Max & Min(array=w128) -> (max value=w127:dbl)  [unwired: 3 out]
    n69 = Index Array(array=w95) -> (element #1=→"슬라이드":waveform(dbl), element #2=→"2":waveform(dbl), element #3=→"슬라이드 2":waveform(dbl), element #4=→"슬라이드 3":waveform(dbl))  [unwired: 4 in]
    n70 = Less?(x=w119, y=0.2) -> (x < y?=w125:bool)
    n71 = Less?(x=w118, y=0.2) -> (x < y?=w124:bool)
    n72 = Greater?(x=w127, y="Force trigger minimum level") -> (0:w126:bool)
    n73 = local read "슬라이드 2"() -> (w100:dbl)
    n74 = local read "슬라이드 3"() -> (w98:dbl)
    n75 = Compound Arithmetic op=AND(w126, w125, w124) -> (w116:bool)
    n76 = local write "trigger"(w116) -> ()
    n77 = local read "슬라이드"() -> (w103:dbl)
    n78 = local read "2"() -> (w99:dbl)
    n79 = Add(x=w103, y=w100) -> (x+y=w112:dbl)
    n80 = Add(x=w99, y=w98) -> (x+y=w109:dbl)
    n81 = Divide(x=w112, y=2.0) -> (x/y=w110:dbl)
    n82 = Divide(x=w109, y=2.0) -> (x/y=w106:dbl)
    n83 = Build Array(w110) -> (w105:dbl[])
    n84 = Build Array(w106) -> (w104:dbl[])
    n85 = Bundle(w105, w104) -> (→"XY 그래프":cluster{dbl[], dbl[]})  [unwired: 1 in]
    n86 = case shown="참" w116 {
      selector: w116 -> [_ w157]
      tunnel: w123 -> [_ w187]
      tunnel: [w141 w155] -> w114
      tunnel: w113 -> [w141 w148]
      frame False {
      }
      frame True {
        w170 = u16 1 items=["인덱스", "시간"] ("location mode")
        w169 = u16 0 items=["하강 에지", "상승 에지"] ("trigger slope")
        w171 = u16 1 items=["인덱스", "시간"] ("location mode")
        w172 = u16 1 items=["하강 에지", "상승 에지"] ("trigger slope")
        w186 = waveform(dbl) {"t0"=timestamp(0 s since 1904-01-01), "dt"=0.00062, "Y"=[]} ("원소")
        n87 = local read "Heater temp 2"() -> (→"Heater temp":dbl)
        n88 = local read "vacum 2"() -> (→"vacum":dbl)
        n89 = case shown="참" "Force cal val" {
          tunnel: [w208 w213] -> w163
          tunnel: [w207 w212] -> w162
          tunnel: [w206 w211] -> w161
          tunnel: [w205 w210] -> w160
          frame False {
            n90 = local read "right mean 4"() -> (w205:dbl)
            n91 = local read "front mean"() -> (w208:dbl)
            n92 = local read "rear mean 3"() -> (w206:dbl)
            n93 = local read "left mean"() -> (w207:dbl)
          }
          frame True {
            (unwired) 0.31 ("y")
            (unwired) 0.39 ("y")
            (unwired) 0.64 ("y")
            (unwired) 0.29 ("y")
            n94 = property on="Strain rear" class="WFChart (엄격한)"() -> ("History Data"=w215:dbl[])  [unwired: 2 in, 2 out]
            n95 = property on="Strain left" class="WFChart (엄격한)"() -> ("History Data"=w214:dbl[])  [unwired: 2 in, 2 out]
            n96 = property on="Strain right" class="WFChart (엄격한)"() -> ("History Data"=w216:dbl[])  [unwired: 2 in, 2 out]
            n97 = property on="Strain front" class="WFChart (엄격한)"() -> ("History Data"=w217:dbl[])  [unwired: 2 in, 2 out]
            n98 = call-poly <vilib>:"Mean.vi"("X"=w217) -> ("mean"=w213:dbl)  [unwired: 1 out]
            n99 = call-poly <vilib>:"Mean.vi"("X"=w214) -> ("mean"=w212:dbl)  [unwired: 1 out]
            n100 = call-poly <vilib>:"Mean.vi"("X"=w215) -> ("mean"=w211:dbl)  [unwired: 1 out]
            n101 = call-poly <vilib>:"Mean.vi"("X"=w216) -> ("mean"=w210:dbl)  [unwired: 1 out]
            n102 = Bundle("mean"=w213, "mean"=w212, "mean"=w211, "mean"=w210) -> (→"strain high level mean":T4)  [unwired: 1 in]
          }
        }
        "front mean" <- w163
        "left mean" <- w162
        "rear mean 3" <- w161
        "right mean 4" <- w160
        n103 = for {
          tunnel: w187 -> [w231] mode=indexing
          shift-right: [w230] -> w177
          shift-left: w186 -> [w225]
          shift-right: [w229] -> w178
          shift-left: w186 -> [w224]
          shift-right: [w228] -> w179
          shift-left: w186 -> [w222]
          shift-right: [w227] -> w180
          shift-left: w186 -> [w219]
          n104 = Index Array(array=w231) -> (element #1=w226:waveform(dbl), element #2=w223:waveform(dbl), element #3=w221:waveform(dbl), element #4=w220:waveform(dbl))  [unwired: 4 in]
          n105 = call-poly <vilib>:"Append Waveforms.vi"("waveform B"=w226, "waveform A"=w225) -> ("waveform out"=w230:waveform(dbl))  [unwired: 8 in, 1 out]
          n106 = call-poly <vilib>:"Append Waveforms.vi"("waveform B"=w223, "waveform A"=w224) -> ("waveform out"=w229:waveform(dbl))  [unwired: 8 in, 1 out]
          n107 = call-poly <vilib>:"Append Waveforms.vi"("waveform B"=w221, "waveform A"=w222) -> ("waveform out"=w228:waveform(dbl))  [unwired: 8 in, 1 out]
          n108 = call-poly <vilib>:"Append Waveforms.vi"("waveform B"=w220, "waveform A"=w219) -> ("waveform out"=w227:waveform(dbl))  [unwired: 8 in, 1 out]
        }
        n109 = call-poly <vilib>:"Amplitude and Levels.vi"("state settings"="state settings", "signal in"=w177) -> ("high state level"=w152:dbl)  [unwired: 6 in, 3 out]
        n110 = call-poly <vilib>:"Amplitude and Levels.vi"("state settings"="state settings", "signal in"=w178) -> ("high state level"=w150:dbl)  [unwired: 6 in, 3 out]
        n111 = call-poly <vilib>:"Amplitude and Levels.vi"("state settings"="state settings", "signal in"=w179) -> ("high state level"=w149:dbl)  [unwired: 6 in, 3 out]
        n112 = call-poly <vilib>:"Amplitude and Levels.vi"("state settings"="state settings", "signal in"=w180) -> ("high state level"=w154:dbl)  [unwired: 6 in, 3 out]
        n113 = Unbundle By Name(w177) -> ("Y"=w182:dbl[])
        n114 = Unbundle By Name(w178) -> ("Y"=w183:dbl[])
        n115 = Unbundle By Name(w179) -> ("Y"=w184:dbl[])
        n116 = Unbundle By Name(w180) -> ("Y"=w185:dbl[])
        n117 = First Call?() -> (First Call?: T/F=w147:bool)
        n118 = Compound Arithmetic op=ADD(w182, w183, w184, w185) -> (w181:dbl[])
        n119 = Or(x=w147, y="reset") -> ()  [unwired: 1 out]
        n120 = case shown="참" "reset" {
          tunnel: w154 -> [w191 w197]
          tunnel: [w191 w196] -> w153
          tunnel: w152 -> [w190 w203]
          tunnel: [w190 w202] -> w151
          tunnel: w150 -> [w189 w200]
          tunnel: [w189 w199] -> w143
          tunnel: w149 -> [w188 w198]
          tunnel: [w188 w201] -> w144
          tunnel: w148 -> [_ w204]
          frame False {
          }
          frame True {
            n121 = Unbundle(w204) -> ("high state level"=w192:dbl, "high state level"=w193:dbl, "high state level"=w194:dbl, "high state level"=w195:dbl)
            n122 = Subtract(x=w192, y=w203) -> (x-y=w202:dbl)
            n123 = Subtract(x=w193, y=w200) -> (x-y=w199:dbl)
            n124 = Subtract(x=w194, y=w198) -> (x-y=w201:dbl)
            n125 = Subtract(x=w195, y=w197) -> (x-y=w196:dbl)
          }
        }
        "level1" <- w151
        "level1 2" <- w143
        "level1 3" <- w144
        "level1 4" <- w153
        "Strain front" <- w151
        "Strain left" <- w143
        "Strain right" <- w153
        "Strain rear" <- w144
        "front" <- w151
        "rear" <- w144
        "left" <- w143
        "right" <- w153
        n126 = Bundle By Name(cluster=w177, "Y"=w181) -> (w145:waveform(dbl))
        "Triggered Force graph" <- w145
        n127 = Bundle("high state level"=w151, "high state level"=w143, "high state level"=w144, "high state level"=w153) -> (w155:T7)  [unwired: 1 in]
        n128 = call-poly <vilib>:"Basic Level Trigger Detection.vi"("signal in"=w145, "level"="bonding time trigger edge level", "location mode"=w171, "trigger slope"=w172) -> ("trigger location"=w167:dbl)  [unwired: 9 in, 2 out]
        "trigger location" <- w167
        n129 = call-poly <vilib>:"Basic Level Trigger Detection.vi"("signal in"=w145, "level"="bonding time trigger edge level", "location mode"=w170, "trigger slope"=w169) -> ("trigger location"=w168:dbl)  [unwired: 9 in, 2 out]
        "trigger location 2" <- w168
        n130 = call-poly <vilib>:"Amplitude and Levels.vi"("state settings"="state settings", "signal in"=w145) -> ("high state level"=→"bonding force" →"웨이브폼 차트 2":dbl)  [unwired: 6 in, 3 out]
        n131 = Subtract(x=w168, y=w167) -> (x-y=→"Bondtime":dbl)
        n132 = Divide(x=w151, y=w163) -> (x/y=w176:dbl)
        n133 = Divide(x=w143, y=w162) -> (x/y=w175:dbl)
        n134 = flat-sequence {
          frame #0 {
            n135 = property on="Filtered force 차트" class="WFChart (엄격한)"("History Data"=waveform(dbl)[][] [[{"t0"=timestamp(0 s since 1904-01-01), "dt"=0.00062, "Y"=[]}]] ("히스토리 데이터")) -> ()  [unwired: 2 in, 2 out]
          }
        }
        n136 = Divide(x=w143, y=w161) -> (x/y=w173:dbl)
        n137 = Divide(x=w153, y=w160) -> (x/y=w174:dbl)
        n138 = Subtract(x=w151, y=w163) -> ()  [unwired: 1 out]
        n139 = Subtract(x=w143, y=w162) -> ()  [unwired: 1 out]
        n140 = Subtract(x=w143, y=w161) -> ()  [unwired: 1 out]
        n141 = Subtract(x=w153, y=w160) -> ()  [unwired: 1 out]
        n142 = Divide(x=w176, y=w175) -> ()  [unwired: 1 out]
        n143 = Divide(x=w173, y=w174) -> ()  [unwired: 1 out]
        "trigger" <- w157
      }
    }
  }
  n144 = call <vilib>:"DAQmx Stop Task.vi"("task/channels in"=w17, "error in"=w18) -> ("task out"=w14:refnum<k21>, "error out"=w15:errorcluster)  [unwired: 12 in]
  n145 = Release Queue(queue=w10, error in (no error)=w8) -> ()  [unwired: 1 in, 3 out]
  n146 = call <vilib>:"DAQmx Clear Task.vi"("task in"=w14, "error in"=w15) -> ()  [unwired: 13 in, 1 out]
